vi "Get Empty Cells with No Neighbours.vi"(0 "Empty Cells":i32[](array[numeric]), 1 "Board Array":T1[](array[typedef])) -> (12 "Empty?":bool, 14 "Intended Array":i32[](array[numeric]), 15 "Empty Cells with Empty Neighbours":i32[](array[numeric]))   [LabVIEW 2014, in "Dragon Tamers.lvlib"]
uses:
  Dragon Tamers.lvlib
  Typedefs/Board Cell.ctl
  Typedefs/Cell Occupancy.ctl
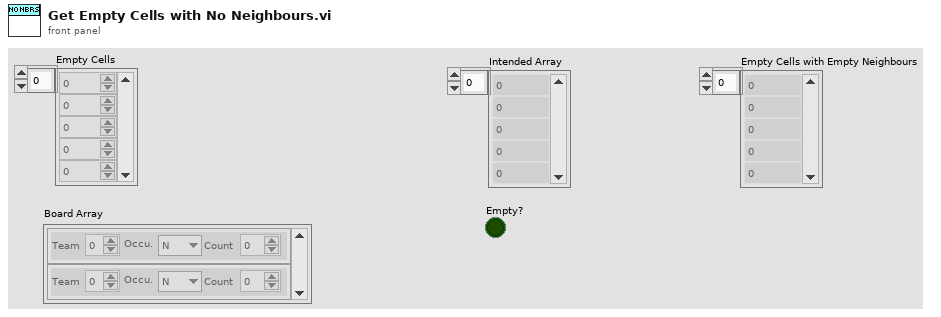
[diagram p1: front panel]
types:
  T1 = typedef "Dragon Tamers.lvlib/Board Cell.ctl" = cluster{"Team":i32, "Occu.":T2, "Count":i32}
  T2 = typedef "Dragon Tamers.lvlib/Cell Occupancy.ctl" = enum16{"N", "C", "K"}
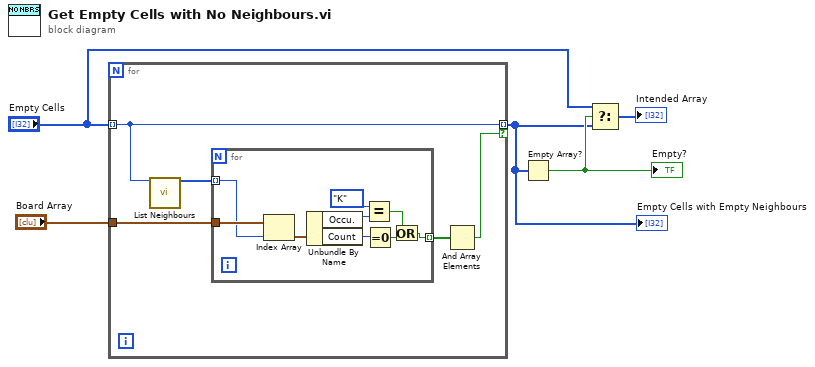
[diagram p0: block diagram]
diagram:
  n1 = for {
    tunnel: "Empty Cells" -> [w7] mode=indexing
    tunnel: "Board Array" -> [w9]
    tunnel: [w7] -> w1 mode=indexing if=w6
    n2 = call "List Neighbours.vi"("Cell Index"=w7) -> ("Neighbours"=w10:i32[])  [unwired: 12 in, 2 out]
    n3 = for {
      tunnel: w10 -> [w16] mode=indexing
      tunnel: w9 -> [w19]
      tunnel: [w11] -> w8 mode=indexing
      n4 = Index Array(array=w19, index=w16) -> (element=w18:T1)
      n5 = Unbundle By Name(w18) -> ("Occu."=w14:T2, "Count"=w17:i32)
      n6 = Equal?(x=Cell_Occupancy."K" ("Occu."), y=w14) -> (x = y?=w12:bool)
      n7 = Equal To 0?(x=w17) -> (x = 0?=w13:bool)
      n8 = Or(x=w12, y=w13) -> (x .or. y?=w11:bool)
    }
    n9 = And Array Elements(Boolean array=w8) -> (logical AND=w6:bool)
  }
  "Empty Cells with Empty Neighbours" <- w1
  n10 = Empty Array?(array=w1) -> (empty?=w4:bool)
  "Empty?" <- w4
  n11 = Select(t="Empty Cells", s=w4, f=w1) -> (s? t:f=→"Intended Array":i32[])
